vi "cRIO AI data3.vi"(6 "Scale factor":dbl, 7 "Chan":i32, 8 "error in (no error)":errorcluster, 10 "Input cluster":T1) -> (0 "error out":errorcluster, 3 "Output":dbl)   [LabVIEW 2020]
panel:
  # "Voltage x factor=actual"
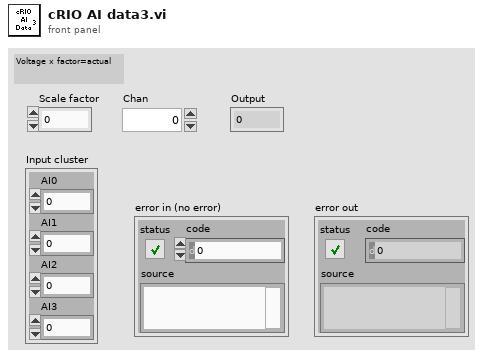
[diagram p1: front panel]
types:
  T1 = cluster{"AI0":dbl, "AI1":dbl, "AI2":dbl, "AI3":dbl}
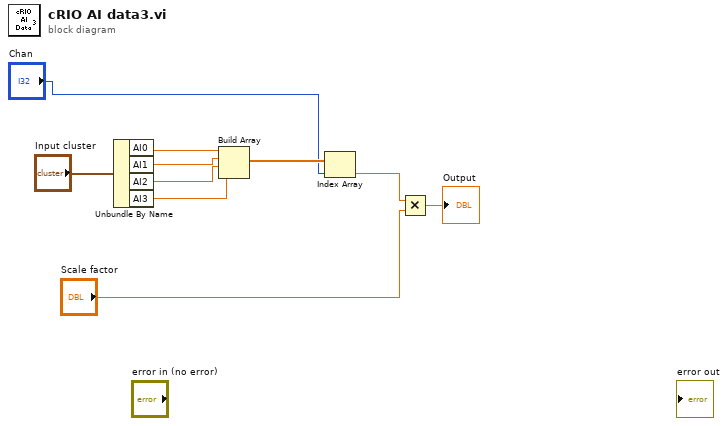
[diagram p0: block diagram]
diagram:
  n1 = Unbundle By Name("Input cluster") -> ("AI0"=w9:dbl, "AI1"=w8:dbl, "AI2"=w7:dbl, "AI3"=w6:dbl)
  n2 = Build Array(w9, w8, w7, w6) -> (w5:dbl[])
  n3 = Index Array(array=w5, index="Chan") -> (element=w3:dbl)
  n4 = Multiply(x=w3, y="Scale factor") -> (x*y=→"Output":dbl)
